vi "myRIO_BRig_Host_TCP_readAccum.vi"(0 "input_strAccum":string, 5 "input_count":i32, 9 "input_handle_TCP":refnum<k5>, 11 "input_error":errorcluster) -> (4 "output_strAccum":string, 6 "output_count":i32, 10 "output_handle_TCP":refnum<k5>, 15 "output_error":errorcluster)   [LabVIEW 2014]
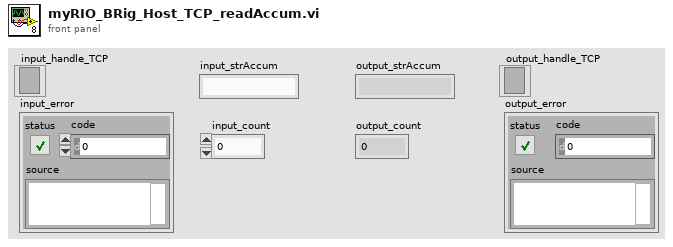
[diagram p1: front panel]
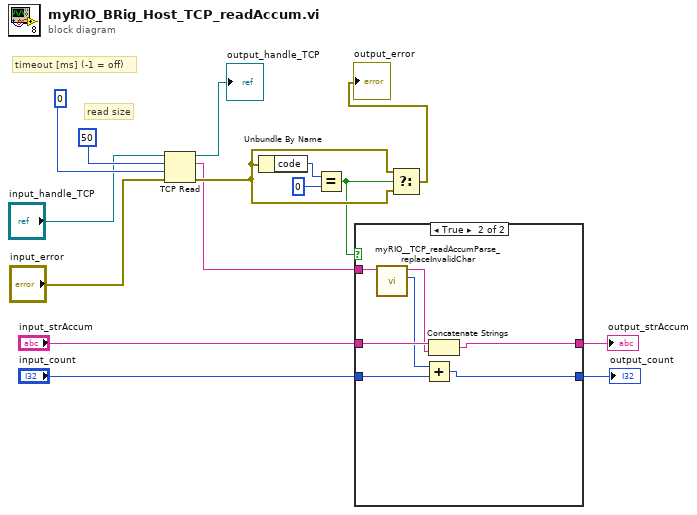
[diagram p0: block diagram]
diagram:
  # "read size"
  # "timeout [ms] (-1 = off)"
  n1 = TCP Read(connection ID="input_handle_TCP", bytes to read=50, error in (no error)="input_error", 9:0 ("timeout ms (25000)")) -> (connection ID out=→"output_handle_TCP":refnum<k5>, data out=w6:string, error out=w8:errorcluster)  [unwired: 1 out]
  n2 = Unbundle By Name(w8) -> ("code"=w10:i32)
  n3 = Equal?(x=w10, y=0) -> (x = y?=w5:bool)
  n4 = case shown="True" w5 {
    tunnel: w6 -> [_ w24]
    tunnel: "input_strAccum" -> [w17 w23]
    tunnel: [w17 w19] -> w3
    tunnel: "input_count" -> [w16 w21]
    tunnel: [w16 w18] -> w1
    frame False {
    }
    frame True {
      n5 = call "myRIO__TCP_readAccumParse_replaceInvalidChar.vi"("input_string"=w24) -> ("output_stringSize"=w20:i32, "output_string"=w22:string)  [unwired: 9 in]
      n6 = Add(x=w20, y=w21) -> (x+y=w18:i32)
      n7 = Concatenate Strings(w23, w22) -> (w19:string)
    }
  }
  "output_strAccum" <- w3
  "output_count" <- w1
  n8 = Select(t=w8, s=w5, f=w8) -> (s? t:f=→"output_error":errorcluster)
